vi "AlazarGetBoardBySystemHandle.vi"(0 "Sys Handle":u64, 1 "Board ID":u32, 2 "error in (no error)":errorcluster) -> (3 "Sys Handle":u64, 4 "Board Handle":u64, 5 "Return Code":u32, 6 "error out":errorcluster)   [LabVIEW 2018]
doc: "Get a handle to a board in a board system where the board system is specified by a handle to its master board, and the board by its identifier within the board system."
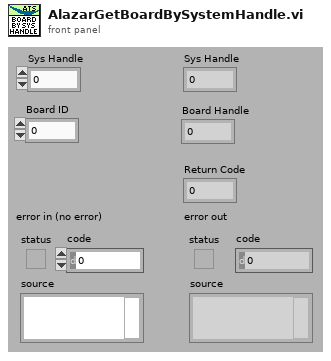
[diagram p1: front panel]
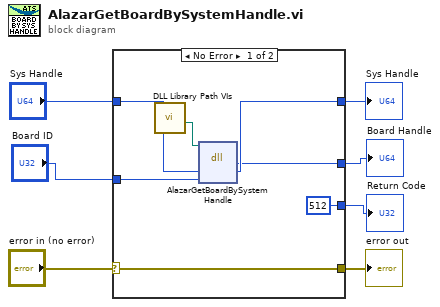
[diagram p0: block diagram]
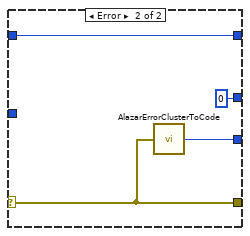
[diagram p2: hidden frame]
diagram:
  n1 = case shown="No Error" "error in (no error)" {
    selector: "error in (no error)" -> [w12 w18]
    tunnel: [w12 w18] -> w6
    tunnel: [u32 512 w17] -> w5
    tunnel: "Sys Handle" -> [w14 w16]
    tunnel: [w13 w16] -> w3
    tunnel: "Board ID" -> [w10 _]
    tunnel: [w9 u32 0] -> w1
    frame No Error {
      n2 = call "DLL Library Path VIs.vi"() -> ("Alazar"=w8:path)  [unwired: 9 in, 2 out]
      n3 = dll-call lib="C:/Project/SerialSectOCT - FFT GPU/SerialSectOCT/Labview Software/DLL/ATSApi.dll" fn="AlazarGetBoardBySystemHandle"(path in=w8, "handle"=w14, "boardId"=w10) -> ("return type"=w9:u64, "handle"=w13:u64)  [unwired: 3 in, 2 out]
    }
    frame Error {
      n4 = call "AlazarErrorClusterToCode.vi"("error in (no error)"=w18) -> ("Error Code"=w17:u32)
    }
  }
  "Sys Handle" <- w3
  "error out" <- w6
  "Return Code" <- w5
  "Board Handle" <- w1
